vi "WPI_DigitalModuleOpen.vi"(8 "error in (no error)":errorcluster) -> (0 "error out":errorcluster, 1 "LoopTiming":u16, 3 "DigitalModuleDevRef":T1)   [LabVIEW 2017]
doc: "This is private and only runs once. Gets an instance of the DIO object for all subsequent digital IO operations.\n\nThis software is licensed. Open the labview\\readme\\WPI Robotics Library Open Source License.txt file for more information."
uses:
  <vilib>/Rock Robotics/WPI/DigitalModule/WPI_DigitalModuleDeviceRef.ctl
  <vilib>/Rock Robotics/SystemInterfaces/System/FPGA_SystemGet.vi
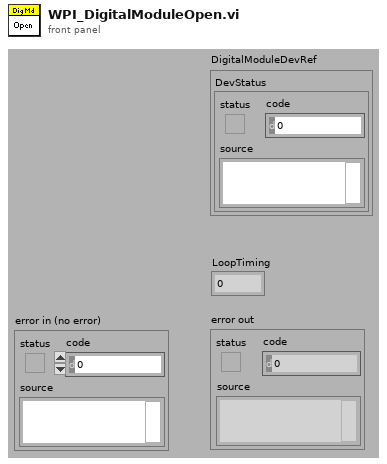
[diagram p1: front panel]
types:
  T1 = typedef "WPI_DigitalModuleDeviceRef.ctl" = cluster{"DevStatus":errorcluster}
  T2 = typedef "FPGA_DIODevRef.ctl" = cluster{"DevStatus":errorcluster}
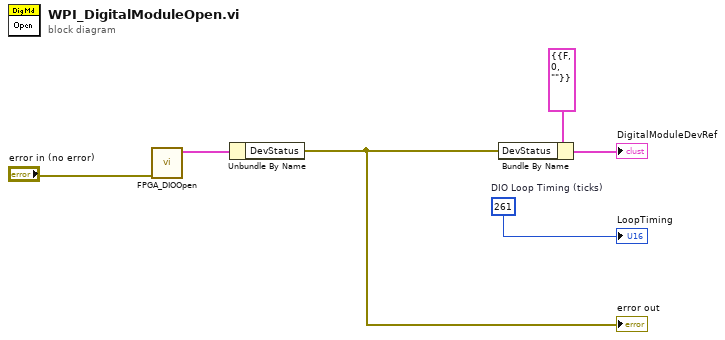
[diagram p0: block diagram]
diagram:
  w1 = u16 261  # DIO Loop Timing (ticks)
  n1 = call <vilib>:"FPGA_DIOOpen.vi"("error in (no error)"="error in (no error)") -> ("DIODeviceRef"=w4:T2)  [unwired: 1 in, 9 out]
  n2 = Unbundle By Name(w4) -> ("DevStatus"=w2:errorcluster)
  "error out" <- w2
  n3 = Bundle By Name(cluster=T1 {"DevStatus"={"status"=FALSE, "code"=0, "source"=""}} ("DigitalModuleDevRef"), "DevStatus"=w2) -> (→"DigitalModuleDevRef":T1)
  "LoopTiming" <- w1
